vi "ImageAveragingFramesv2.vi"(0 "y-index":i32, 5 "x pix":i32, 7 "Frames grabbed":i32, 9 "Frames to grab (grab)":i32, 11 "Images 3D in":dbl[][][](array[numeric]), 12 "new":dbl[](array[numeric])) -> (4 "Images 3D out":dbl[][][](array[numeric]), 6 "Images 2D out":dbl[][](array[numeric]))   [LabVIEW 2012, in "Image.lvclass"]
uses:
  classes/Image.lvclass
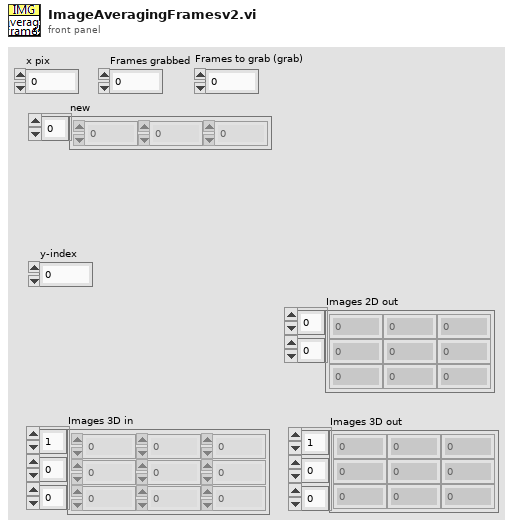
[diagram p1: front panel]
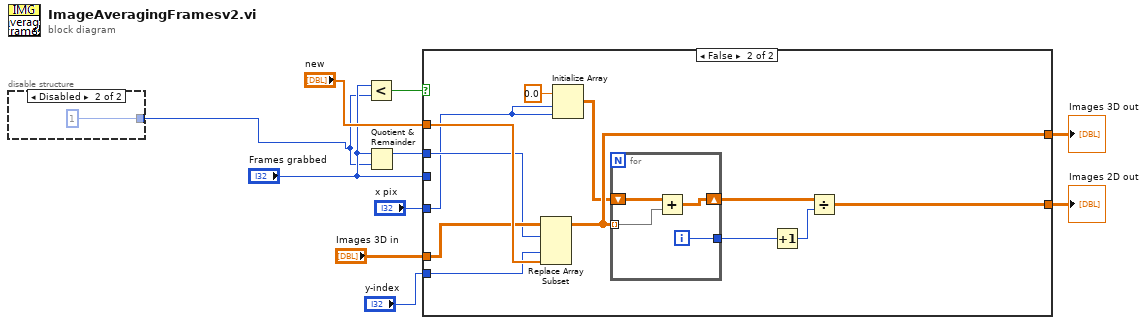
[diagram p0: block diagram]
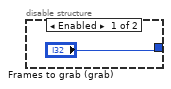
[diagram p2: hidden frame]
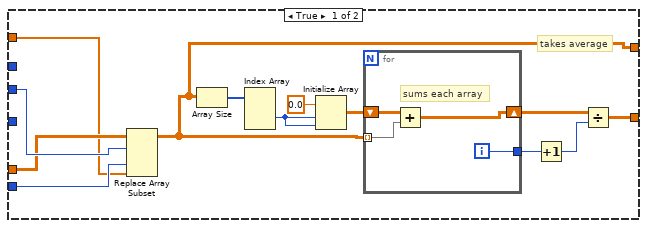
[diagram p3: hidden frame]
diagram:
  n1 = disable-structure shown="Disabled" {
    disable-tunnel: ["Frames to grab (grab)" 1] -> w1
    frame Enabled {
    }
    frame Disabled {
    }
  }
  n2 = Less?(x="Frames grabbed", y=w1) -> (x < y?=w2:bool)
  n3 = Quotient & Remainder(x="Frames grabbed", y=w1) -> (x-y*floor(x/y)=w6:i32)  [unwired: 1 out]
  n4 = case shown="False" w2 {
    tunnel: "Images 3D in" -> [w14 w34]
    tunnel: "Frames grabbed" -> [w17 _]
    tunnel: "new" -> [w13 w41]
    tunnel: "y-index" -> [w16 w40]
    tunnel: [w15 w35] -> w8
    tunnel: [w25 w38] -> w7
    tunnel: w6 -> [_ w33]
    tunnel: "x pix" -> [_ w31]
    frame True {
      # "takes average"
      n5 = Replace Array Subset(array=w14, new element=w13, index (dim 0)=w17, index (dim 2)=w16) -> (w15:dbl[][][])  [unwired: 1 in]
      n6 = Array Size(array=w15) -> (size(s)=w19:i32[])
      n7 = Index Array(array=w19) -> (element #2=w18:i32)  [unwired: 3 in, 2 out]
      n8 = Initialize Array(0.0 ("element"), w18, w18) -> (w22:dbl[][])
      n9 = for {
        shift-right: [w29] -> w24
        shift-left: w22 -> [w28]
        tunnel: [w27] -> w21
        tunnel: w15 -> [w26] mode=indexing
        i -> [w27]
        # "sums each array"
        n10 = Add(x=w28, y=w26) -> (x+y=w29:dbl[][])
      }
      n11 = Increment(x=w21) -> (x+1=w20:i32)
      n12 = Divide(x=w24, y=w20) -> (x/y=w25:dbl[][])
    }
    frame False {
      n13 = Replace Array Subset(array=w34, new element=w41, index (dim 0)=w33, index (dim 2)=w40) -> (w35:dbl[][][])  [unwired: 1 in]
      n14 = Initialize Array(0.0 ("element"), w31, w31) -> (w30:dbl[][])
      n15 = for {
        shift-right: [w45] -> w39
        shift-left: w30 -> [w44]
        tunnel: [w43] -> w37
        tunnel: w35 -> [w42] mode=indexing
        i -> [w43]
        n16 = Add(x=w44, y=w42) -> (x+y=w45:dbl[][])
      }
      n17 = Increment(x=w37) -> (x+1=w36:i32)
      n18 = Divide(x=w39, y=w36) -> (x/y=w38:dbl[][])
    }
  }
  "Images 2D out" <- w7
  "Images 3D out" <- w8
